vi "data_minMax.vi"(8 "error in (no error)":errorcluster, 9 "AcqData":sgl[](array[numeric]) format="%.2f", 10 "length":i32, 11 "idx start":i32) -> (0 "error out":errorcluster, 1 "dataOut":sgl[](array[numeric]), 2 "min":sgl, 3 "max":sgl)   [LabVIEW 2010, in "OSA.lvclass"]
uses:
  OSA.lvclass
  OSA20X_misc.lvlib
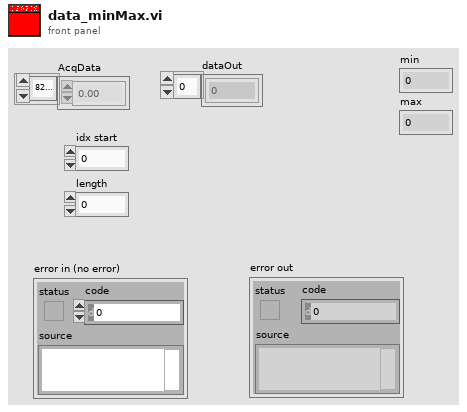
[diagram p1: front panel]
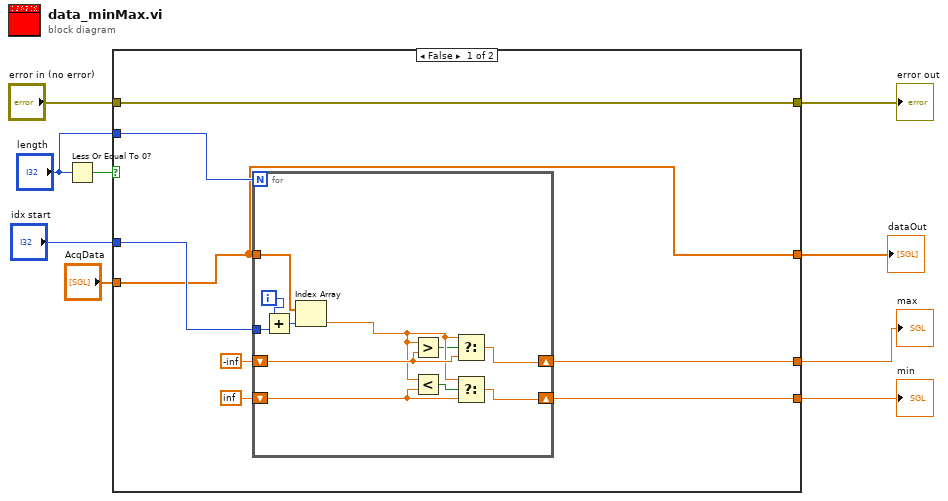
[diagram p0: block diagram]
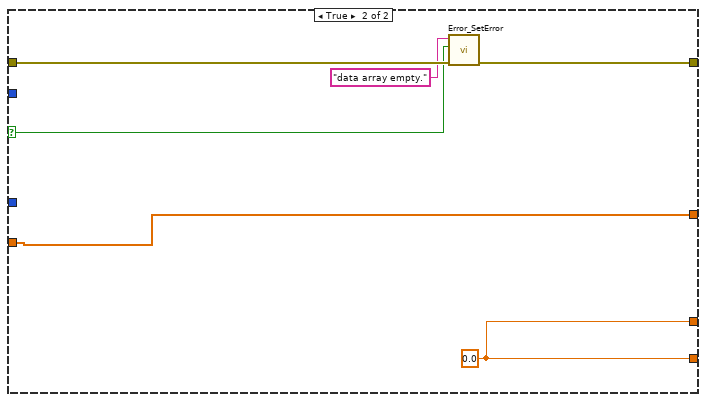
[diagram p2: hidden frame]
diagram:
  n1 = Less Or Equal To 0?(x="length") -> (x <= 0?=w6:bool)
  n2 = case shown="False" w6 {
    selector: w6 -> [_ w32]
    tunnel: [w17 w34] -> w9
    tunnel: [w16 w34] -> w8
    tunnel: "idx start" -> [w13 _]
    tunnel: "error in (no error)" -> [w10 w33]
    tunnel: [w10 w30] -> w4
    tunnel: "AcqData" -> [w11 w29]
    tunnel: [w11 w29] -> w2
    tunnel: "length" -> [w12 _]
    frame False {
      n3 = for {
        N: w12 -> [_]
        shift-right: [w27] -> w16
        shift-left: sgl -inf -> [w28]
        shift-right: [w25] -> w17
        shift-left: sgl inf -> [w26]
        tunnel: w13 -> [w20]
        tunnel: w11 -> [w18]
        i -> [w21]
        n4 = Add(x=w21, y=w20) -> (x+y=w19:i32)
        n5 = Index Array(array=w18, index=w19) -> (element=w24:sgl)
        n6 = Greater?(x=w24, y=w28) -> (0:w23:bool)
        n7 = Less?(x=w24, y=w26) -> (x < y?=w22:bool)
        n8 = Select(t=w24, s=w23, f=w28) -> (s? t:f=w27:sgl)
        n9 = Select(t=w24, s=w22, f=w26) -> (s? t:f=w25:sgl)
      }
    }
    frame True {
      w34 = sgl 0.0
      n10 = call "Error_SetError.vi"("error in"=w33, "status (true)"=w32, "source(\"\")"="data array empty." ("source(\"\")")) -> ("error out"=w30:errorcluster)  [unwired: 4 in]
    }
  }
  "min" <- w9
  "max" <- w8
  "error out" <- w4
  "dataOut" <- w2
